vi "attackTacticCheckStateChange.vi"(8 "error in (no error)":errorcluster, 9 "Robot In":refnum<class "Robot.lvclass">, 10 "Game in":refnum<class "Game.lvclass">, 11 "AttackTacticVSS in":refnum<class "AttackTacticVSS.lvclass">) -> (0 "error out":errorcluster, 2 "State":enum16{"Kick", "Exit", "GoToBall", "BallToGoal"}(ring), 3 "AttackTacticVSS out":refnum<class "AttackTacticVSS.lvclass">)   [LabVIEW 2023, in "AttackTacticVSS.lvclass"]
uses:
  AttackTacticVSS.lvclass
  Game_class/Game.lvclass
  Robot_class/Robot.lvclass
  C:/Users/roboi/Downloads/VSS_AI-Larc2023 - Copia (2)/Object_class/Object.lvclass
  Utilities_class/Utilities.lvclass
  Game_class/Game.lvclass/Game.ctl
  Object_class/Object.lvclass/Object.ctl
  Object_class/Read x.vi
  Object_class/Read y.vi
  Game_class/Read BallRef.vi
  Game_class/Read EnemyRef.vi
  Game_class/Read FieldRef.vi
  Ball_class/Ball.lvclass
  Enemy_class/Enemy.lvclass
  Field_class/Field.lvclass
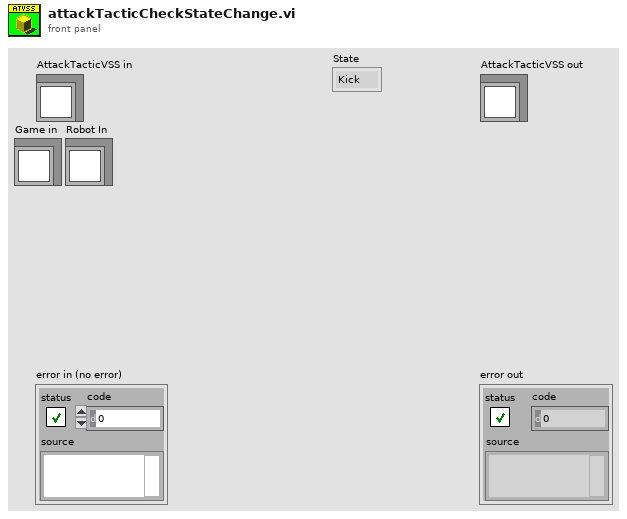
[diagram p1: front panel]
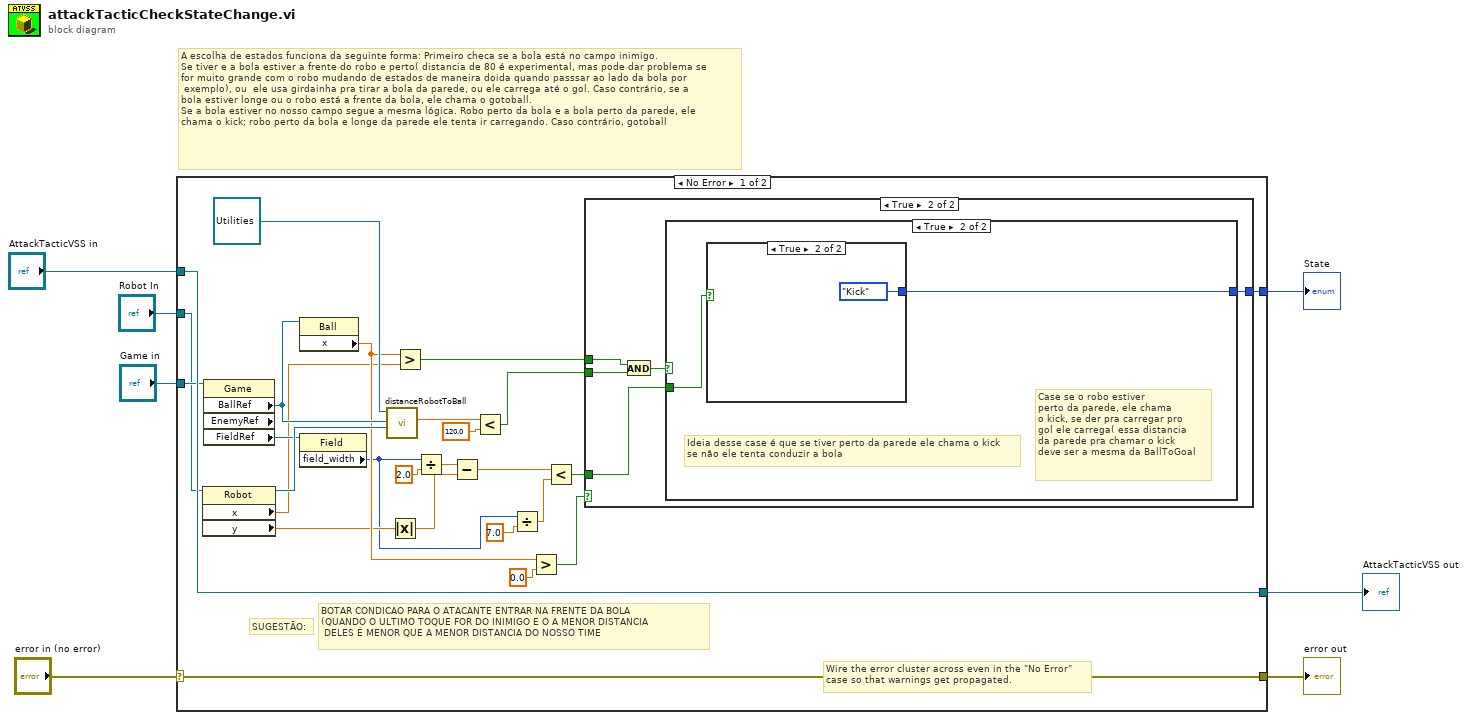
[diagram p0: block diagram]
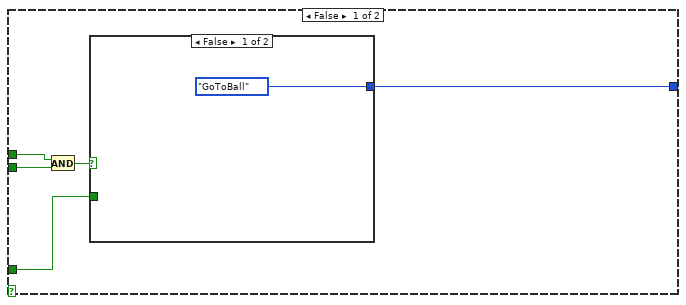
[diagram p2: hidden frame]
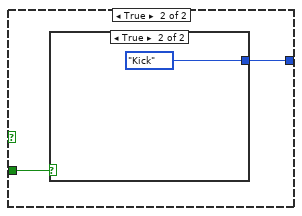
[diagram p3: hidden frame]
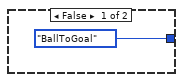
[diagram p4: hidden frame]
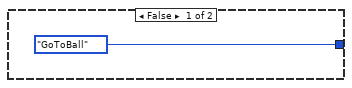
[diagram p5: hidden frame]
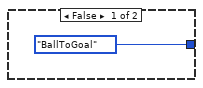
[diagram p6: hidden frame]
diagram:
  # "A escolha de estados funciona da seguinte forma: Primeiro checa se a bola está no campo inimigo. \nSe tiver e a bola estiver a frente do robo e perto( distancia de 80 é experimental, mas pode dar problema se\nfor muito grande com o robo mudando de estados de maneira doida quando passsar ao lado da bola por\n exemplo), ou  ele usa girdainha pra tirar a bola da parede, ou ele carrega até o gol. Caso contrário, se a \nbola estiver longe ou o robo está a frente da bola, ele chama o gotoball. \nSe a bola estiver no nosso campo segue a mesma lógica. Robo perto da bola e a bola perto da parede, ele \nchama o kick; robo perto da bola e longe da parede ele tenta ir carregando. Caso contrário, gotoball"
  n1 = case shown="No Error" "error in (no error)" {
    selector: "error in (no error)" -> [w32 w55]
    tunnel: [w32 w55] -> w6
    tunnel: [w33 w54] -> w4
    tunnel: "AttackTacticVSS in" -> [w33 w54]
    tunnel: "Game in" -> [w31 _]
    tunnel: "Robot In" -> [w28 _]
    tunnel: [w21 _] -> w1
    frame No Error {
      # "SUGESTÃO:"
      # "BOTAR CONDICAO PARA O ATACANTE ENTRAR NA FRENTE DA BOLA\n(QUANDO O ULTIMO TOQUE FOR DO INIMIGO E O A MENOR DISTANCIA\n DELES É MENOR QUE A MENOR DISTANCIA DO NOSSO TIME"
      # "Wire the error cluster across even in the \"No Error\"\ncase so that warnings get propagated."
      n2 = property class="Robot"(reference=w28) -> (reference out=w29:refnum<class "Robot.lvclass">, "x"=w16:dbl, "y"=w11:dbl)  [unwired: 1 in, 1 out]
      n3 = property class="Game" props=["BallRef", "EnemyRef", "FieldRef"](reference=w31) -> ("BallRef"=w27:refnum<class "Ball.lvclass">, "FieldRef"=w18:refnum<class "Field.lvclass">)  [unwired: 1 in, 3 out]
      n4 = property class="Ball"(reference=w27) -> ("x"=w20:dbl)  [unwired: 1 in, 2 out]
      n5 = property class="Field"(reference=w18) -> ("field_width"=w10:i32)  [unwired: 1 in, 2 out]
      n6 = call "distanceRobotToBall.vi"("Robot"=w29, "Ball"=w27, "Utilities in"=refnum<class "Utilities.lvclass"> refnum) -> ("Distance Robot To Ball"=w24:dbl)  [unwired: 6 in, 2 out]
      n7 = Absolute Value(x=w11) -> (abs(x)=w14:dbl)
      n8 = Greater?(x=w20, y=w16) -> (0:w19:bool)
      n9 = Divide(x=w10, y=2.0) -> (x/y=w15:dbl)
      n10 = Subtract(x=w15, y=w14) -> (x-y=w13:dbl)
      n11 = Less?(x=w24, y=120.0) -> (x < y?=w22:bool)
      n12 = Divide(x=w10, y=7.0) -> (x/y=w8:dbl)
      n13 = Greater?(x=w20, y=0.0) -> (0:w25:bool)
      n14 = Less?(x=w13, y=w8) -> (x < y?=w12:bool)
      n15 = case shown="True" w25 {
        tunnel: w22 -> [w37 w46]
        tunnel: [w38 w48] -> w21
        tunnel: w19 -> [w36 w47]
        tunnel: w12 -> [w34 w44]
        frame False {
          n16 = And(x=w36, y=w37) -> (x .and. y?=w35:bool)
          n17 = case shown="False" w35 {
            tunnel: [enum16{"Kick", "Exit", "GoToBall", "BallToGoal"}."GoToBall" ("State") w41] -> w38
            tunnel: w34 -> [_ w40]
            frame False {
            }
            frame True {
              n18 = case shown="True" w40 {
                tunnel: [enum16{"Kick", "Exit", "GoToBall", "BallToGoal"}."BallToGoal" ("State") enum16{"Kick", "Exit", "GoToBall", "BallToGoal"}."Kick" ("State")] -> w41
                frame False {
                }
                frame True {
                }
              }
            }
          }
        }
        frame True {
          n19 = And(x=w47, y=w46) -> (x .and. y?=w45:bool)
          n20 = case shown="True" w45 {
            tunnel: [enum16{"Kick", "Exit", "GoToBall", "BallToGoal"}."GoToBall" ("State") w50] -> w48
            tunnel: w44 -> [_ w51]
            frame False {
            }
            frame True {
              # "Ideia desse case é que se tiver perto da parede ele chama o kick\nse não ele tenta conduzir a bola"
              # "Case se o robo estiver\nperto da parede, ele chama\no kick, se der pra carregar pro\ngol ele carrega( essa distancia\nda parede pra chamar o kick\ndeve ser a mesma da BallToGoal"
              n21 = case shown="True" w51 {
                tunnel: [enum16{"Kick", "Exit", "GoToBall", "BallToGoal"}."BallToGoal" ("State") enum16{"Kick", "Exit", "GoToBall", "BallToGoal"}."Kick" ("State")] -> w50
                frame False {
                }
                frame True {
                }
              }
            }
          }
        }
      }
    }
    frame Error {
    }
  }
  "error out" <- w6
  "AttackTacticVSS out" <- w4
  "State" <- w1
